vi "heartbeat.vi"(8 "error in (no error)":errorcluster, 11 "AlCS in":refnum<class "AlCS.lvclass">) -> (0 "error out":errorcluster, 1 "newValue":bool, 2 "answer":string, 3 "AlCS out":refnum<class "AlCS.lvclass">)   [LabVIEW 2016, in "AlCS.lvclass"]
uses:
  AlCS.lvclass
  AlCS.lvclass/AlCS.ctl
  Heartbeat/Heartbeat.lvclass
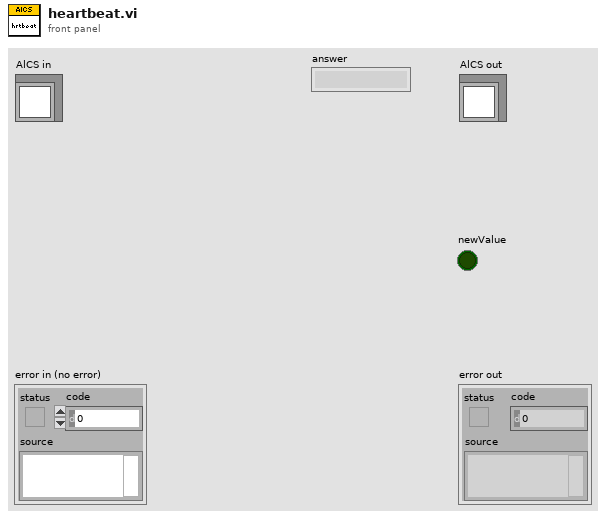
[diagram p1: front panel]
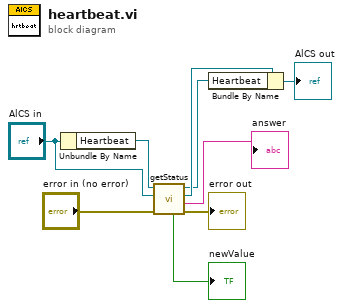
[diagram p0: block diagram]
diagram:
  n1 = Unbundle By Name("AlCS in") -> ("Heartbeat"=w9:refnum<class "Heartbeat.lvclass">)
  n2 = call "getStatus.vi"("error in (no error)"="error in (no error)", "AlCS in"="AlCS in", "Heartbeat in"=w9) -> ("error out"=→"error out":errorcluster, "answer"=→"answer":string, "AlCS out"=w7:refnum<class "AlCS.lvclass">, "Heartbeat out"=w6:refnum<class "Heartbeat.lvclass">, "newValue"=→"newValue":bool)  [unwired: 4 in]
  n3 = Bundle By Name(cluster=w7, "Heartbeat"=w6) -> (→"AlCS out":refnum<class "AlCS.lvclass">)
